vi "CountingFPGA.vi"() -> ()   [LabVIEW 2016]
uses:
  <vilib>/rvi/Emulation/niFpgaGetClockAttributes.vi
  <vilib>/rvi/Emulation/niFpgaSctlEmulationGetInTimedLoop.vi
  <vilib>/rvi/Emulation/niFpgaEmulationReportErrorSimple.vi
  <vilib>/rvi/Emulation/niFpgaProcessEmulError.vi
  <vilib>/rvi/Emulation/niFpgaCriticalErrorInLSC.vi
  <vilib>/rvi/eio/common/nirviEmuTemplateMethod_errors.vi
  <vilib>/eio/EIONode/EIONode.xnode
panel:
  out "stop if true":bool
  in  "ZERO HL":fxp<+,18,3>
  in  "THR HL":fxp<+,18,3>
  in  "ZERO HR":fxp<+,18,3>
  in  "THR HR":fxp<+,18,3>
  out "vHL":sgl
  out "vHR":sgl
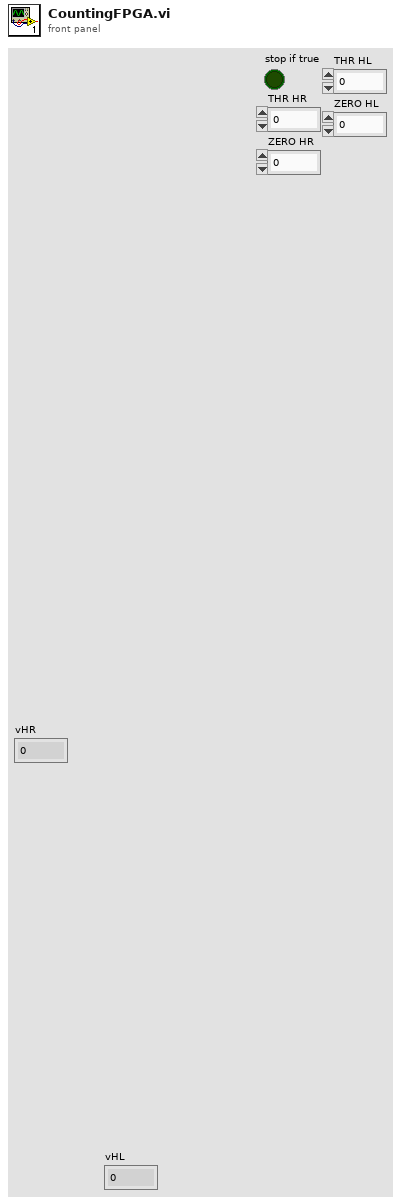
[diagram p1: front panel]
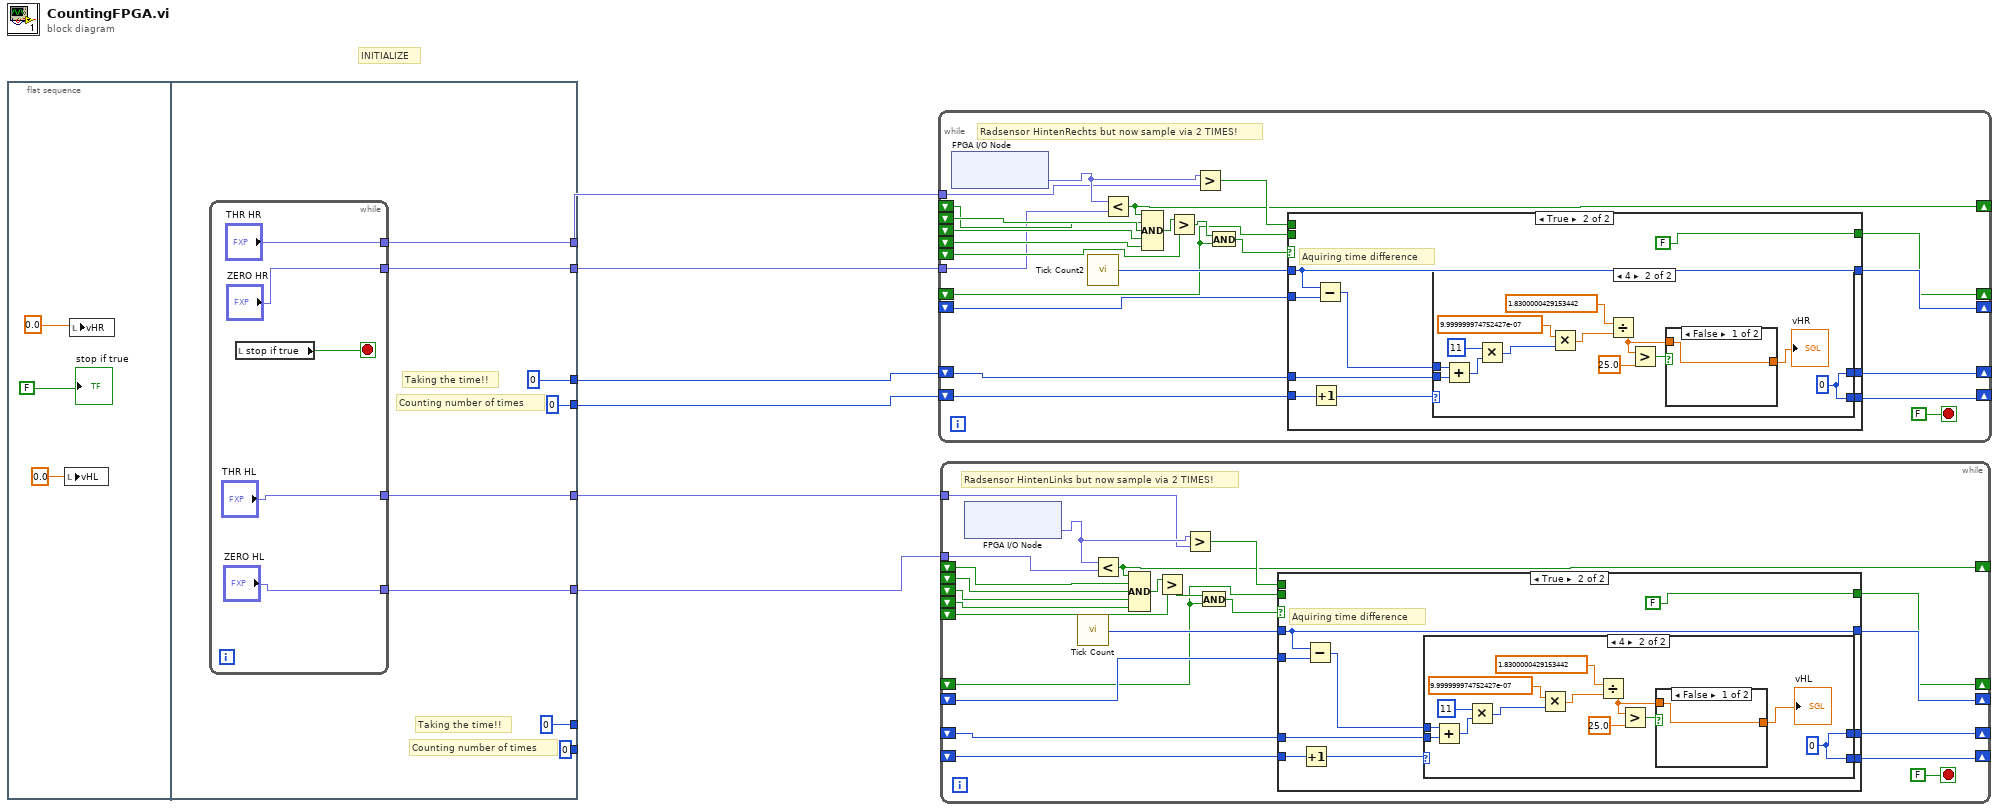
[diagram p0: block diagram]
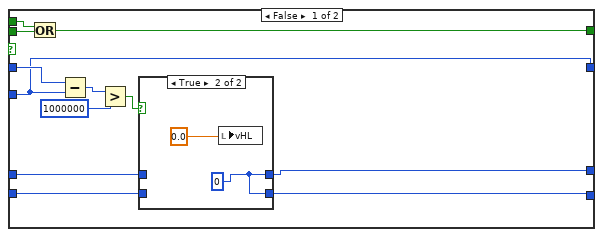
[diagram p2: hidden frame]
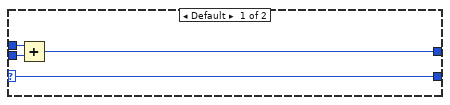
[diagram p4: hidden frame]
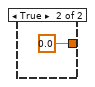
[diagram p5: hidden frame]
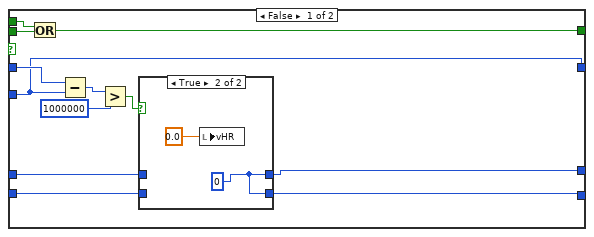
[diagram p6: hidden frame]
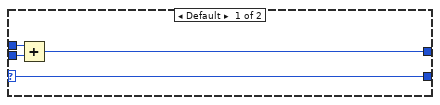
[diagram p8: hidden frame]
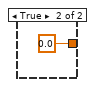
[diagram p9: hidden frame]
diagram:
  # "INITIALIZE"
  n1 = flat-sequence {
    tunnel: [i16 0] -> _
    tunnel: [i16 0] -> _
    tunnel: [i16 0] -> w6
    tunnel: [i16 0] -> w5
    tunnel: [w11] -> w4
    tunnel: [w10] -> w3
    tunnel: [w13] -> w2
    tunnel: [w12] -> w1
    frame #0 {
      n2 = local write "vHL"(sgl 0.0) -> ()
      n3 = local write "vHR"(sgl 0.0) -> ()
      "stop if true" <- FALSE
    }
    frame #1 {
      # "Taking the time!!"
      # "Counting number of times"
      # "Taking the time!!"
      # "Counting number of times"
      n4 = while {
        tunnel: ["THR HR"] -> w13
        tunnel: ["ZERO HR"] -> w12
        tunnel: ["THR HL"] -> w11
        tunnel: ["ZERO HL"] -> w10
        stop <- w18 stop-if-true
        n5 = local read "stop if true"() -> (w18:bool)
      }
    }
  }
  n6 = while {
    shift-right: [w31] -> _
    shift-left: _ -> [w25]
    shift-right: [w43] -> _
    shift-left: _ -> [w42]
    shift-right: [w41] -> _
    shift-left: w5 -> [w40]
    shift-right: [w39] -> _
    shift-left: w6 -> [w38]
    shift-right: [w33] -> _
    shift-left: _ -> [w34]
    shift-left: _ -> [w26]
    shift-left: _ -> [w27]
    shift-left: _ -> [w28]
    shift-left: _ -> [w29]
    tunnel: w2 -> [w24]
    tunnel: w1 -> [w23]
    stop <- FALSE stop-if-true
    # "Radsensor HintenRechts but now sample via 2 TIMES!"
    n7 = xnode "FPGA I/O Node"() -> ("Mod2/AI0"=w32:fxp<+,18,3>)  [unwired: 1 in, 1 out]
    n8 = call "Tick Count2"() -> ("Tick Count(uSec)"=w44:u32)
    n9 = Less?(x=w32, y=w23) -> (x < y?=w31:bool)
    n10 = Compound Arithmetic op=AND(w31, w25, w26, w27, w28) -> (w30:bool)
    n11 = Greater?(x=w30, y=w29) -> (0:w37:bool)
    n12 = Greater?(x=w32, y=w24) -> (0:w35:bool)
    n13 = And(x=w37, y=w34) -> (x .and. y?=w36:bool)
    n14 = case shown="True" w36 {
      tunnel: w44 -> [w54 w70]
      tunnel: [w53 w70] -> w43
      tunnel: w42 -> [w53 w69]
      tunnel: w40 -> [w47 w68]
      tunnel: [w46 w66] -> w41
      tunnel: w38 -> [w49 w65]
      tunnel: [w48 w63] -> w39
      tunnel: w35 -> [w57 _]
      tunnel: w34 -> [w56 _]
      tunnel: [w55 FALSE] -> w33
      frame False {
        n15 = Or(x=w57, y=w56) -> (x .or. y?=w55:bool)
        n16 = Subtract(x=w54, y=w53) -> (x-y=w51:u32)
        n17 = Greater?(x=w51, y=u32 1000000) -> (0:w52:bool)
        n18 = case shown="True" w52 {
          tunnel: w49 -> [w59 _]
          tunnel: [w59 w61] -> w48
          tunnel: w47 -> [w58 _]
          tunnel: [w58 w61] -> w46
          frame False {
          }
          frame True {
            w61 = 0
            n19 = local write "vHR"(sgl 0.0) -> ()
          }
        }
      }
      frame True {
        # "Aquiring time difference"
        n20 = Increment(x=w68) -> (x+1=w67:i32)
        n21 = Subtract(x=w70, y=w69) -> (x-y=w64:u32)
        n22 = case shown="4" w67 {
          selector: w67 -> [w74 _]
          tunnel: [w74 w87] -> w66
          tunnel: w65 -> [w73 w86]
          tunnel: w64 -> [w72 w85]
          tunnel: [w71 w87] -> w63
          frame Default {
            n23 = Add(x=w72, y=w73) -> (x+y=w71:u32)
          }
          frame 4 {
            w87 = i16 0
            n24 = Add(x=w85, y=w86) -> (x+y=w84:u32)
            n25 = Multiply(x=u32 11, y=w84) -> (x*y=w81:u32)
            n26 = Multiply(x=sgl 1e-06, y=w81) -> (x*y=w79:sgl)
            n27 = Divide(x=sgl 1.83, y=w79) -> (x/y=w77:sgl)
            n28 = Greater?(x=w77, y=sgl 25.0) -> (0:w76:bool)
            n29 = case shown="False" w76 {
              tunnel: w77 -> [w88 _]
              tunnel: [w88 sgl 0.0] -> w75
              frame False {
              }
              frame True {
              }
            }
            "vHR" <- w75
          }
        }
      }
    }
  }
  n30 = while {
    shift-right: [w96] -> _
    shift-left: _ -> [w95]
    shift-right: [w110] -> _
    shift-left: _ -> [w109]
    shift-right: [w108] -> _
    shift-left: _ -> [w107]
    shift-right: [w106] -> _
    shift-left: _ -> [w105]
    shift-right: [w100] -> _
    shift-left: _ -> [w101]
    shift-left: _ -> [w94]
    shift-left: _ -> [w93]
    shift-left: _ -> [w92]
    shift-left: _ -> [w98]
    tunnel: w4 -> [w91]
    tunnel: w3 -> [w90]
    stop <- FALSE stop-if-true
    # "Radsensor HintenLinks but now sample via 2 TIMES!"
    n31 = xnode "FPGA I/O Node"() -> ("Mod2/AI1"=w99:fxp<+,18,3>)  [unwired: 1 in, 1 out]
    n32 = call "Tick Count"() -> ("Tick Count(uSec)"=w111:u32)
    n33 = Less?(x=w99, y=w90) -> (x < y?=w96:bool)
    n34 = Compound Arithmetic op=AND(w96, w95, w94, w93, w92) -> (w97:bool)
    n35 = Greater?(x=w97, y=w98) -> (0:w104:bool)
    n36 = Greater?(x=w99, y=w91) -> (0:w102:bool)
    n37 = And(x=w104, y=w101) -> (x .and. y?=w103:bool)
    n38 = case shown="True" w103 {
      tunnel: w111 -> [w121 w137]
      tunnel: [w120 w137] -> w110
      tunnel: w109 -> [w120 w136]
      tunnel: w107 -> [w114 w135]
      tunnel: [w113 w133] -> w108
      tunnel: w105 -> [w116 w132]
      tunnel: [w115 w130] -> w106
      tunnel: w102 -> [w124 _]
      tunnel: w101 -> [w123 _]
      tunnel: [w122 FALSE] -> w100
      frame False {
        n39 = Or(x=w124, y=w123) -> (x .or. y?=w122:bool)
        n40 = Subtract(x=w121, y=w120) -> (x-y=w118:u32)
        n41 = Greater?(x=w118, y=u32 1000000) -> (0:w119:bool)
        n42 = case shown="True" w119 {
          tunnel: w116 -> [w126 _]
          tunnel: [w126 w128] -> w115
          tunnel: w114 -> [w125 _]
          tunnel: [w125 w128] -> w113
          frame False {
          }
          frame True {
            w128 = 0
            n43 = local write "vHL"(sgl 0.0) -> ()
          }
        }
      }
      frame True {
        # "Aquiring time difference"
        n44 = Increment(x=w135) -> (x+1=w134:i32)
        n45 = Subtract(x=w137, y=w136) -> (x-y=w131:u32)
        n46 = case shown="4" w134 {
          selector: w134 -> [w141 _]
          tunnel: [w141 w154] -> w133
          tunnel: w132 -> [w140 w153]
          tunnel: w131 -> [w139 w152]
          tunnel: [w138 w154] -> w130
          frame Default {
            n47 = Add(x=w139, y=w140) -> (x+y=w138:u32)
          }
          frame 4 {
            w154 = i16 0
            n48 = Add(x=w152, y=w153) -> (x+y=w151:u32)
            n49 = Multiply(x=u32 11, y=w151) -> (x*y=w148:u32)
            n50 = Multiply(x=sgl 1e-06, y=w148) -> (x*y=w146:sgl)
            n51 = Divide(x=sgl 1.83, y=w146) -> (x/y=w144:sgl)
            n52 = Greater?(x=w144, y=sgl 25.0) -> (0:w143:bool)
            n53 = case shown="False" w143 {
              tunnel: w144 -> [w155 _]
              tunnel: [w155 sgl 0.0] -> w142
              frame False {
              }
              frame True {
              }
            }
            "vHL" <- w142
          }
        }
      }
    }
  }
